vi "UsrProfiles-Parse param names.vi"(10 "key":string, 11 "Saved value":dbl) -> (3 "String":string)   [LabVIEW 2017]
uses:
  Typedefs/Movement mode.ctl
  Typedefs/Channel Selector.ctl
  Typedefs/Line draw mode.ctl
  Typedefs/Imaging Protocols enum.ctl
  Typedefs/AOL modes.ctl
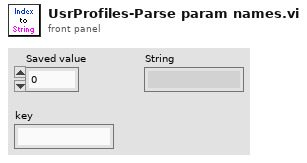
[diagram p1: front panel]
types:
  T1 = typedef "Movement mode.ctl" = enum16{"Move the frame", "Move the feature"}
  T2 = typedef "Channel Selector.ctl" = enum16{"Red Channel", "Green Channel", "Blended"}
  T3 = enum16{"Grayscale", "Binary", "Gradient", "Rainbow", "Temperature", "User Defined"}
  T4 = typedef "Line draw mode.ctl" = enum16{"Free draw", "Orthogonal"}
  T5 = typedef "Imaging Protocols enum.ctl" = enum16{"AOL Z-Stack", "Motor Z Stack", "Functional Acquisition", "Single Plane Acquisition", "Volume Acquisition", "Live Imaging", "Live Plane Imaging", "Live Volume Imaging"}
  T6 = typedef "AOL modes.ctl" = enum16{"Raster", "Structural", "Pointing", "Mini Scan", "Alignment"}
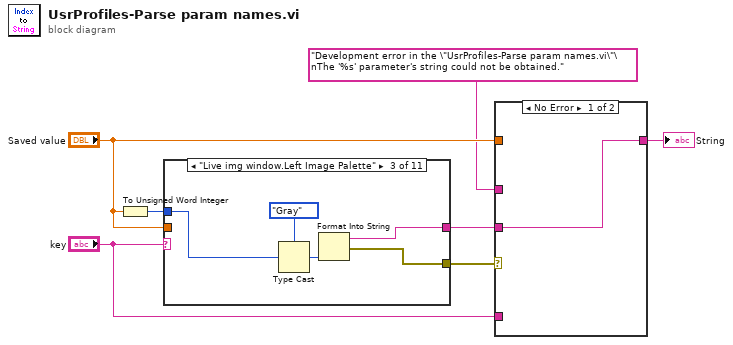
[diagram p0: block diagram]
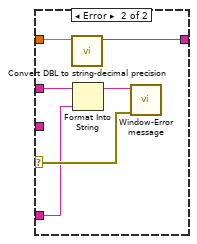
[diagram p2: hidden frame]
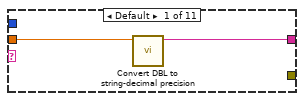
[diagram p3: hidden frame]
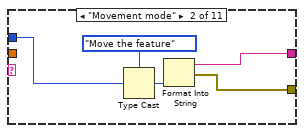
[diagram p4: hidden frame]
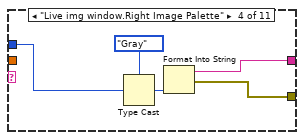
[diagram p5: hidden frame]
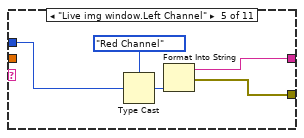
[diagram p6: hidden frame]
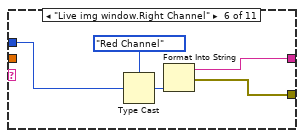
[diagram p7: hidden frame]
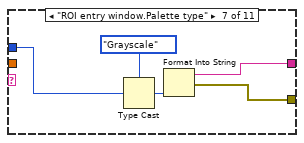
[diagram p8: hidden frame]
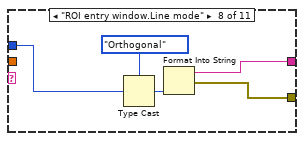
[diagram p9: hidden frame]
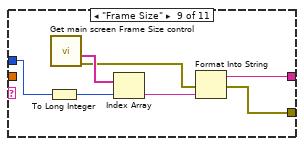
[diagram p10: hidden frame]
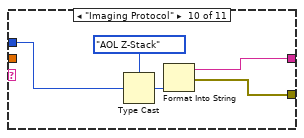
[diagram p11: hidden frame]
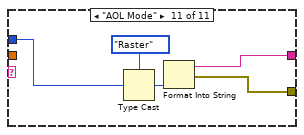
[diagram p12: hidden frame]
diagram:
  n1 = To Unsigned Word Integer(number="Saved value") -> (unsigned 16bit integer=w7:u16)
  n2 = case shown="\"Live img window.Left Image Palette\"" "key" {
    tunnel: w7 -> [_ w14 w19 w24 w29 w34 w39 w44 w49 w56 w61]
    tunnel: [w8 w11 w17 w22 w27 w32 w37 w42 w51 w54 w59] -> w4
    tunnel: [_ w10 w16 w21 w26 w31 w36 w41 w50 w53 w58] -> w6
    tunnel: "Saved value" -> [w9 _ _ _ _ _ _ _ _ _ _]
    frame Default {
      n3 = call <userlib>:"Convert DBL to string-decimal precision.vi"("DBL Value"=w9) -> ("Converted to String"=w8:string)  [unwired: 10 in]
    }
    frame "Movement mode" {
      n4 = Type Cast(type=Movement_mode."Move the feature" ("Movement mode"), x=w14) -> (*(type *) &x=w13:T1)
      n5 = Format Into String(w13) -> (resulting string=w11:string, error out=w10:errorcluster)  [unwired: 3 in]
    }
    frame "Live img window.Left Image Palette" {
      n6 = Type Cast(type=enum16{"Gray", "Red", "Green"}."Gray" ("Value"), x=w19) -> (*(type *) &x=w18:enum16{"Gray", "Red", "Green"})
      n7 = Format Into String(w18) -> (resulting string=w17:string, error out=w16:errorcluster)  [unwired: 3 in]
    }
    frame "Live img window.Right Image Palette" {
      n8 = Type Cast(type=enum16{"Gray", "Red", "Green"}."Gray" ("Value"), x=w24) -> (*(type *) &x=w23:enum16{"Gray", "Red", "Green"})
      n9 = Format Into String(w23) -> (resulting string=w22:string, error out=w21:errorcluster)  [unwired: 3 in]
    }
    frame "Live img window.Left Channel" {
      n10 = Type Cast(type=Channel_Selector."Red Channel" ("Value"), x=w29) -> (*(type *) &x=w28:T2)
      n11 = Format Into String(w28) -> (resulting string=w27:string, error out=w26:errorcluster)  [unwired: 3 in]
    }
    frame "Live img window.Right Channel" {
      n12 = Type Cast(type=Channel_Selector."Red Channel" ("Value"), x=w34) -> (*(type *) &x=w33:T2)
      n13 = Format Into String(w33) -> (resulting string=w32:string, error out=w31:errorcluster)  [unwired: 3 in]
    }
    frame "ROI entry window.Palette type" {
      n14 = Type Cast(type=T3."Grayscale" ("Value"), x=w39) -> (*(type *) &x=w38:T3)
      n15 = Format Into String(w38) -> (resulting string=w37:string, error out=w36:errorcluster)  [unwired: 3 in]
    }
    frame "ROI entry window.Line mode" {
      n16 = Type Cast(type=Line_draw_mode."Orthogonal" ("Value"), x=w44) -> (*(type *) &x=w43:T4)
      n17 = Format Into String(w43) -> (resulting string=w42:string, error out=w41:errorcluster)  [unwired: 3 in]
    }
    frame "Frame Size" {
      n18 = To Long Integer(number=w49) -> (32bit integer=w48:i32)
      n19 = call "Get main screen Frame Size control.vi"() -> ("error out"=w45:errorcluster, "Strings []"=w46:string[])  [unwired: 9 in, 1 out]
      n20 = Index Array(array=w46, index=w48) -> (element=w47:string)
      n21 = Format Into String(error in=w45, w47) -> (resulting string=w51:string, error out=w50:errorcluster)  [unwired: 2 in]
    }
    frame "Imaging Protocol" {
      n22 = Type Cast(type=Imaging_Protocols_enum."AOL Z-Stack" ("Imaging Protocol"), x=w56) -> (*(type *) &x=w55:T5)
      n23 = Format Into String(w55) -> (resulting string=w54:string, error out=w53:errorcluster)  [unwired: 3 in]
    }
    frame "AOL Mode" {
      n24 = Type Cast(type=AOL_modes."Raster" ("AOL Mode"), x=w61) -> (*(type *) &x=w60:T6)
      n25 = Format Into String(w60) -> (resulting string=w59:string, error out=w58:errorcluster)  [unwired: 3 in]
    }
  }
  n26 = case shown="No Error" w6 {
    selector: w6 -> [_ w64]
    tunnel: "Saved value" -> [_ w68]
    tunnel: w4 -> [w62 _]
    tunnel: [w62 w67] -> w3
    tunnel: "Development error in the \"UsrProfiles-Parse param names.vi\"\nThe '%s' parameter's string could not be obtained." ("Message") -> [_ w66]
    tunnel: "key" -> [_ w63]
    frame No Error {
    }
    frame Error {
      n27 = call <userlib>:"Convert DBL to string-decimal precision.vi"("DBL Value"=w68) -> ("Converted to String"=w67:string)  [unwired: 10 in]
      n28 = Format Into String(initial string=w66, w63) -> (resulting string=w65:string)  [unwired: 2 in, 1 out]
      n29 = call "Window-Error message.vi"("error in (no error)"=w64, "Message"=w65) -> ()  [unwired: 9 in, 1 out]
    }
  }
  "String" <- w3
